vi "BuildMenu5.vi"(0 "XRef":T16, 1 "MenuRef":T15, 2 "Point":T13, 3 "Menu Type":T12, 4 "State In":T2) -> (14 "Fatal Error Out":T1)   [LabVIEW 2020, in "Parallel Diagram Block.xnode"]
uses:
  Parallel Diagram Block.xnode
  <vilib>/XNodeSupport/XNodeInt.ctl
  <vilib>/XNodeSupport/NI_XNodeSupport.lvlib
  Parallel Block/OpMenu Action.ctl
  Parallel Block/Parallel Block.lvlib
  <vilib>/XNodeSupport/XNodeXNodeRef.ctl
  <vilib>/XNodeSupport/XNodeMenuRef.ctl
  <vilib>/XNodeSupport/XNodePoint.ctl
  <vilib>/XNodeSupport/XNodeMenuType.ctl
  <vilib>/XNodeSupport/XNodeErrorCluster.ctl
  State.ctl
  Parallel Block/Value Type.ctl
  Parallel Block/Type Descriptor.ctl
  <vilib>/picture/picture.llb/imagedata.ctl
  Parallel Block/Direction.ctl
  Parallel Block/Terminal Mode.ctl
  Parallel Block/Terminal Type.ctl
  Parallel Block/Type Mode.ctl
  Parallel Block/Value Mode.ctl
  Parallel Block/Manager Node.ctl
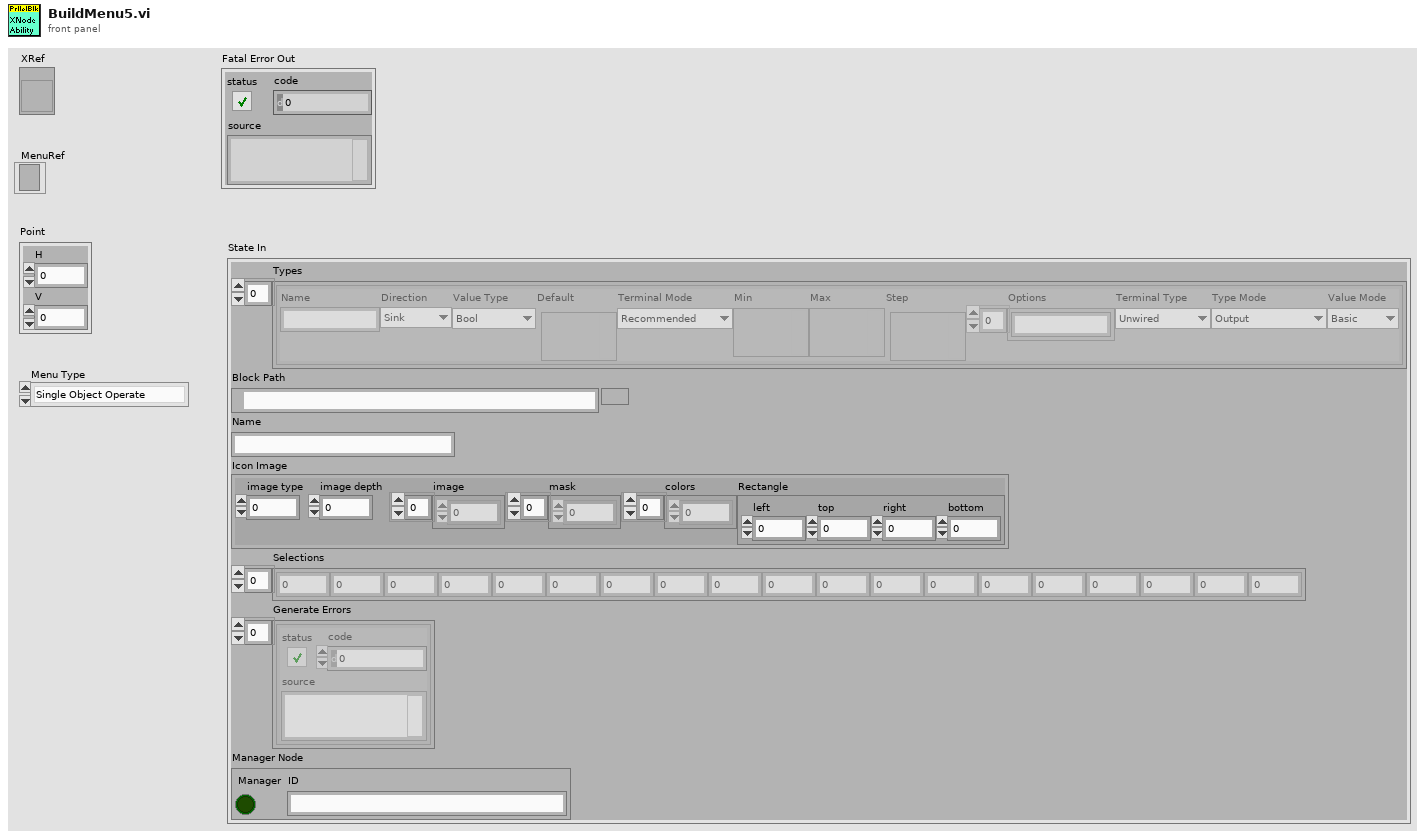
[diagram p1: front panel]
types:
  T1 = typedef "NI_XNodeSupport.lvlib/XNodeErrorCluster.ctl" = errorcluster
  T2 = typedef "Parallel Diagram Block.xnode/State.ctl" = cluster{"Types":T3[], "Block Path":path, "Name":string, "Icon Image":T10, "Selections":i32[], "Generate Errors":errorcluster[], "Manager Node":T11}
  T3 = typedef "Parallel Block.lvlib/Type Descriptor.ctl" = cluster{"Name":string, "Direction":T4, "Value Type":T5, "Default":variant, "Terminal Mode":T6, "Min":variant, "Max":variant, "Step":variant, "Options":string[], "Terminal Type":T7, "Type Mode":T8, "Value Mode":T9}
  T4 = typedef "Parallel Block.lvlib/Direction.ctl" = enum16{"Sink", "Source"}
  T5 = typedef "Parallel Block.lvlib/Value Type.ctl" = enum16{"Unknown", "Bool", "U8", "U16", "U32", "U64", "I8", "I16", "I32", "I64", "SGL", "DBL", "CSG", "CDB", "CDBWfm", "String", "DBLWfm"}
  T6 = typedef "Parallel Block.lvlib/Terminal Mode.ctl" = enum16{"Recommended", "Required", "None"}
  T7 = typedef "Parallel Block.lvlib/Terminal Type.ctl" = enum16{"Unwired", "BadType", "Connection", "Value", "Control Ref", "BadRefType"}
  T8 = typedef "Parallel Block.lvlib/Type Mode.ctl" = enum16{"Output", "Single - Strict", "Single - Coerced", "Stream"}
  T9 = typedef "Parallel Block.lvlib/Value Mode.ctl" = enum16{"Basic", "Range", "Select"}
  T10 = typedef "imagedata.ctl" = cluster{"image type":i32, "image depth":i32, "image":u8[], "mask":u8[], "colors":u32[], "Rectangle":cluster{"left":i16, "top":i16, "right":i16, "bottom":i16}}
  T11 = typedef "Parallel Block.lvlib/Manager Node.ctl" = cluster{"Manager":bool, "ID":string}
  T12 = typedef "NI_XNodeSupport.lvlib/XNodeMenuType.ctl" = enum32{"Single Object Operate", "Single Object Popup", "Multi Object Popup Master", "Multi Object Popup Other"}
  T13 = typedef "NI_XNodeSupport.lvlib/XNodePoint.ctl" = cluster{"H":T14, "V":T14}
  T14 = typedef "NI_XNodeSupport.lvlib/XNodeInt.ctl" = i32
  T15 = typedef "NI_XNodeSupport.lvlib/XNodeMenuRef.ctl" = refnum<k9>
  T16 = typedef "NI_XNodeSupport.lvlib/XNodeXNodeRef.ctl" = refnum<vi>
  T17 = typedef "Parallel Block.lvlib/OpMenu Action.ctl" = enum16{"Selector"}
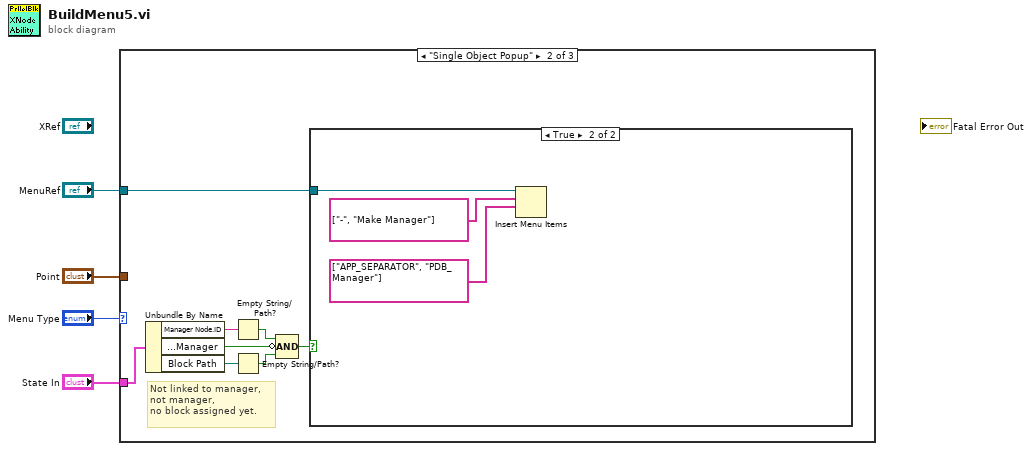
[diagram p0: block diagram]
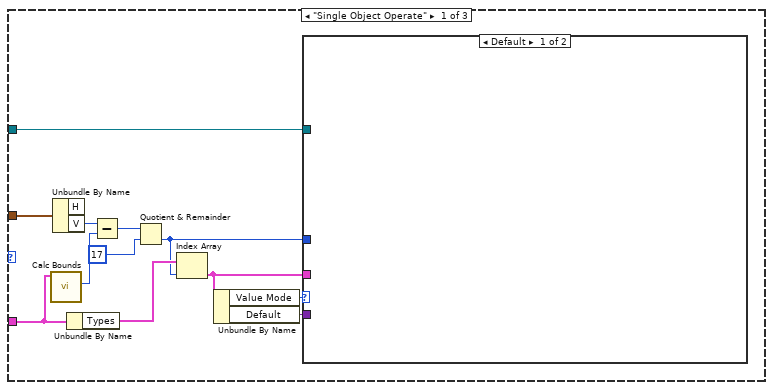
[diagram p2: hidden frame]
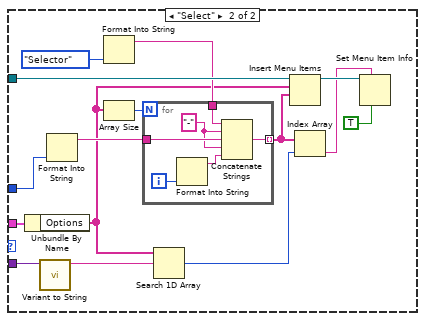
[diagram p3: hidden frame]
diagram:
  n1 = case shown="\"Single Object Popup\"" "Menu Type" {
    tunnel: "State In" -> [w6 w45 _]
    tunnel: "Point" -> [w11 _ _]
    tunnel: "MenuRef" -> [w8 w38 _]
    frame "Single Object Operate" {
      n2 = call "Calc Bounds.vi"("State"=w6) -> ("Header"=w15:i32)  [unwired: 4 in, 6 out]
      n3 = Unbundle By Name(w11) -> ("V"=w16:T14)  [unwired: 1 out]
      n4 = Unbundle By Name(w6) -> ("Types"=w12:T3[])
      n5 = Subtract(x=w16, y=w15) -> (x-y=w14:T14)
      n6 = Quotient & Remainder(x=w14, y=T14 17) -> (floor(x/y)=w7:T14)  [unwired: 1 out]
      n7 = Index Array(array=w12, index=w7) -> (element=w9:T3)
      n8 = Unbundle By Name(w9) -> ("Value Mode"=w10:T9, "Default"=w5:variant)
      n9 = case shown="Default" w10 {
        tunnel: w9 -> [_ w31]
        tunnel: w8 -> [_ w27]
        tunnel: w7 -> [_ w30]
        tunnel: w5 -> [_ w23]
        frame Default {
        }
        frame "Select" {
          n10 = Unbundle By Name(w31) -> ("Options"=w21:string[])
          n11 = call "Variant to String.vi"("Value"=w23) -> ("String"=w22:string)  [unwired: 10 in]
          n12 = Format Into String(w30) -> (resulting string=w29:string)  [unwired: 3 in, 1 out]
          n13 = Format Into String(OpMenu_Action."Selector" ("OpMenu Action")) -> (resulting string=w25:string)  [unwired: 3 in, 1 out]
          n14 = Array Size(array=w21) -> (size(s)=w28:i32)
          n15 = for {
            N: w28 -> [_]
            tunnel: w29 -> [w36]
            tunnel: [w34] -> w20 mode=indexing
            tunnel: w25 -> [w32]
            i -> [w37]
            w33 = "-" ("string")
            n16 = Format Into String(w37) -> (resulting string=w35:string)  [unwired: 3 in, 1 out]
            n17 = Concatenate Strings(w32, w33, w36, w33, w35) -> (w34:string)
          }
          n18 = Search 1D Array(1D array=w21, element=w22) -> (index of element=w19:i32)  [unwired: 1 in]
          n19 = Insert Menu Items(7:w20, 8:w21, 9:w27) -> (3:w24:refnum<k9>)  [unwired: 3 in, 2 out]
          n20 = Index Array(array=w20, index=w19) -> (element=w18:string)
          n21 = Set Menu Item Info(6:TRUE ("checked"), 7:w18, 11:w24) -> ()  [unwired: 4 in, 2 out]
        }
      }
    }
    frame "Single Object Popup" {
      # "Not linked to manager,\nnot manager,\nno block assigned yet."
      n22 = Unbundle By Name(w45) -> ("Manager Node.ID"=w41:string, "Manager Node.Manager"=w43:bool, "Block Path"=w44:path)
      n23 = Empty String/Path?(string/path=w41) -> (empty?=w40:bool)
      n24 = Empty String/Path?(string/path=w44) -> (empty?=w42:bool)
      n25 = Compound Arithmetic op=AND(w40, invert w43, w42) -> (w39:bool)
      n26 = case shown="True" w39 {
        tunnel: w38 -> [_ w48]
        frame False {
        }
        frame True {
          n27 = Insert Menu Items(7:string[] ["APP_SEPARATOR", "PDB_Manager"] ("item names"), 8:string[] ["-", "Make Manager"] ("item names"), 9:w48) -> ()  [unwired: 3 in, 3 out]
        }
      }
    }
    frame Default {
    }
  }
